vi "Write VISA resource name.vi"(8 "error in (no error)":errorcluster, 10 "VISA resource name":refnum<visa-resource-name>, 11 "Agilent 34401a in":refnum<class "Agilent 34401a.lvclass">) -> (0 "error out":errorcluster, 3 "Agilent 34401a out":refnum<class "Agilent 34401a.lvclass">)   [LabVIEW 2013, in "Agilent 34401a.lvclass"]
uses:
  Agilent 34401a.lvclass
  Agilent 34401a.lvclass/Agilent 34401a.ctl
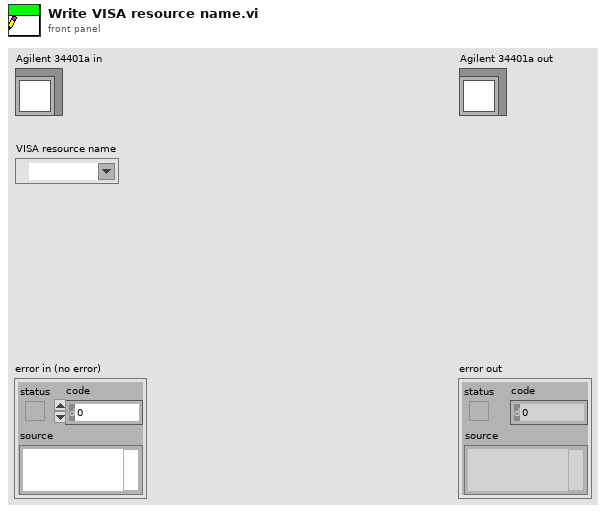
[diagram p1: front panel]
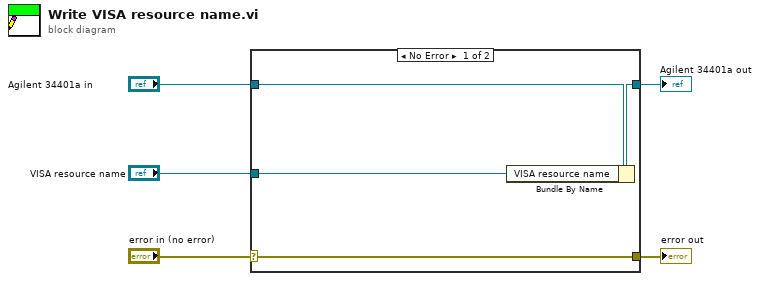
[diagram p0: block diagram]
diagram:
  n1 = case shown="No Error" "error in (no error)" {
    selector: "error in (no error)" -> [w9 w10]
    tunnel: [w9 w10] -> w4
    tunnel: [w7 w11] -> w2
    tunnel: "Agilent 34401a in" -> [w8 w11]
    tunnel: "VISA resource name" -> [w6 _]
    frame No Error {
      n2 = Bundle By Name(cluster=w8, "VISA resource name"=w6) -> (w7:refnum<class "Agilent 34401a.lvclass">)
    }
    frame Error {
    }
  }
  "error out" <- w4
  "Agilent 34401a out" <- w2
